vi "Calibration_File_Path_Subvi.vi"(10 "Enum":T1(ring)=enum."Flywheel") -> (2 "File Path":string)   [LabVIEW 2019]
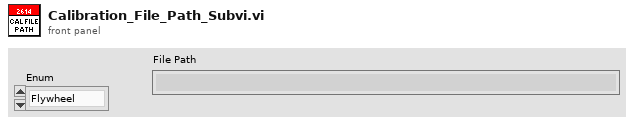
[diagram p1: front panel]
types:
  T1 = enum16{"Turret", "Magazine", "Intake", "Flywheel", "Drive", "Climb"}
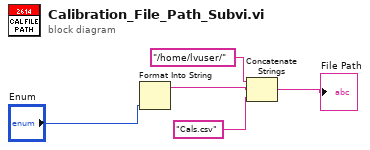
[diagram p0: block diagram]
diagram:
  n1 = Format Into String("Enum") -> (resulting string=w4:string)  [unwired: 3 in, 1 out]
  n2 = Concatenate Strings("/home/lvuser/", w4, "Cals.csv") -> (→"File Path":string)
